vi "Read_Image(Batch).vi"(5 "mBatch":i32, 6 "PreProcessing_Options":T1={"DS_Name"="", "Input_Dims"={"C"=0, "H"=224, "W"=224}, "Center Crop Size"=-1, "Interpolation Type"=1, "Multi-Stage_DownSample?"=FALSE, "Dataset_Stats"={"means"={"R"=0.5385, "G"=0.5348, "B"=0.551}, "stds"={"R"=0.3673, "G"=0.3673, "B"=0.3505}}} {"Dataset_Stats"."stds"."R" format="%#_3g"; "Dataset_Stats"."stds"."G" format="%#_3g"; "Dataset_Stats"."stds"."B" format="%#_3g"; "Dataset_Stats"."means"."R" format="%#_3g"; "Dataset_Stats"."means"."G" format="%#_3g"; "Dataset_Stats"."means"."B" format="%#_3g"; "Interpolation Type" items=["Zero Order", "Bi-Linear", "Quadratic", "Cubic Spline"]}, 8 "error in":errorcluster, 9 "index":i32, 11 "Array":path[][](array[path])) -> (0 "error out":errorcluster, 2 "dT_Img_Read":dbl format="%0.2f", 3 "Image(Batch) Out":sgl[][][][](array[numeric]))   [LabVIEW 2020]
uses:
  <vilib>/Analysis/NI_AALBase.lvlib
  <vilib>/Analysis/baseanly.llb/Mean (DBL).vi
  <vilib>/Ngene/DeepLTK Anomaly Detection Addon/DeepLTK_Anomaly_Detection_Addon/API/Controls/NNPC_DS_Stats.ctl
  <vilib>/Ngene/DeepLTK Anomaly Detection Addon/DeepLTK_Anomaly_Detection_Addon/DeepLTK_Anomaly_Detection_Addon.lvlib
  <vilib>/Ngene/Deep Learning Toolkit/Toolkit/NN_Data/API/NN_Dims(C,H,W).ctl
  <vilib>/Ngene/Deep Learning Toolkit/Toolkit/Deep_Learning_Toolkit_by_Ngene.lvlib
  <vilib>/Ngene/DeepLTK Anomaly Detection Addon/DeepLTK_Anomaly_Detection_Addon/API/Controls/NNPC_PreProcessing_Options.ctl
  <vilib>/Ngene/DeepLTK Anomaly Detection Addon/DeepLTK_Anomaly_Detection_Addon/API/Controls/Image_Stats_RGB.ctl
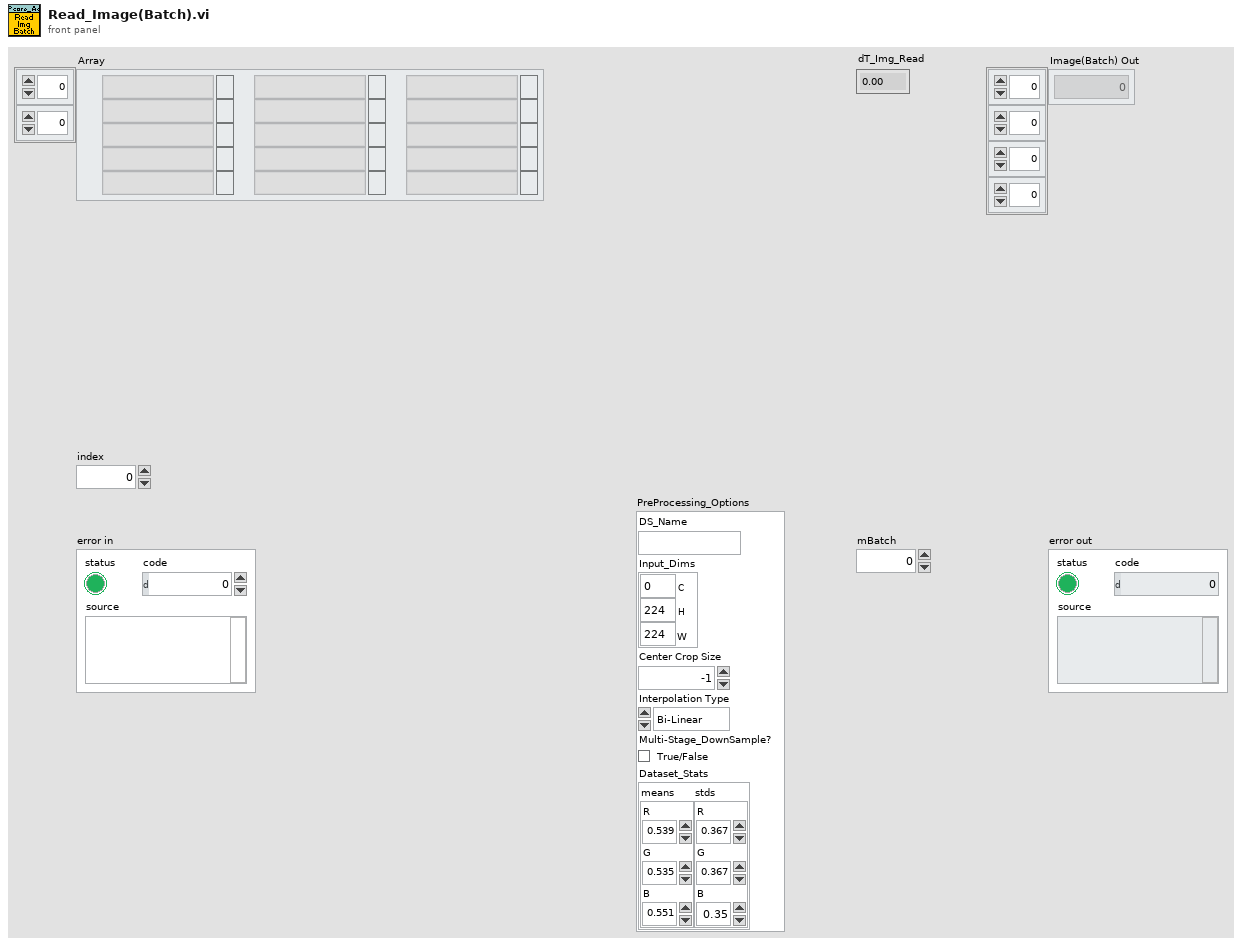
[diagram p1: front panel]
types:
  T1 = typedef "DeepLTK_Anomaly_Detection_Addon.lvlib/NNPC_PreProcessing_Options.ctl" = cluster{"DS_Name":string, "Input_Dims":T2, "Center Crop Size":i32, "Interpolation Type":u32, "Multi-Stage_DownSample?":bool, "Dataset_Stats":T3}
  T2 = typedef "Deep_Learning_Toolkit_by_Ngene.lvlib/NN_Dims(C,H,W).ctl" = cluster{"C":i32, "H":i32, "W":i32}
  T3 = typedef "DeepLTK_Anomaly_Detection_Addon.lvlib/NNPC_DS_Stats.ctl" = cluster{"means":T4, "stds":T4}
  T4 = typedef "DeepLTK_Anomaly_Detection_Addon.lvlib/Image_Stats_RGB.ctl" = cluster{"R":sgl, "G":sgl, "B":sgl}
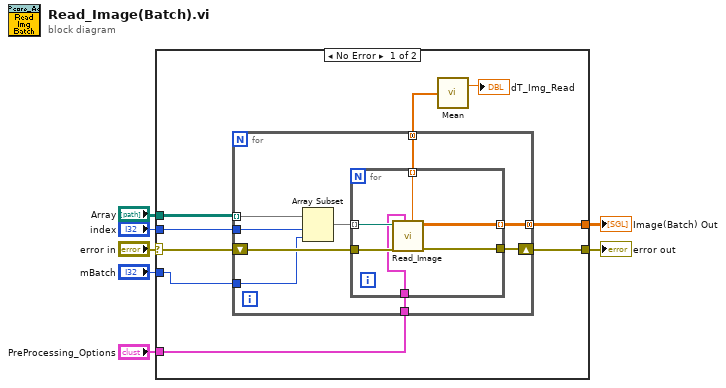
[diagram p0: block diagram]
diagram:
  n1 = case shown="No Error" "error in" {
    selector: "error in" -> [w9 w32]
    tunnel: [w16 _] -> w7
    tunnel: [w15 w32] -> w6
    tunnel: "Array" -> [w14 _]
    tunnel: "PreProcessing_Options" -> [w13 _]
    tunnel: "index" -> [w12 _]
    tunnel: "mBatch" -> [w8 _]
    frame No Error {
      n2 = for {
        tunnel: [w24] -> w11 mode=concatenating
        tunnel: w14 -> [w19] mode=indexing
        tunnel: [w23] -> w16 mode=concatenating
        tunnel: w13 -> [w21]
        shift-right: [w22] -> w15
        shift-left: w9 -> [w25]
        tunnel: w12 -> [w18]
        tunnel: w8 -> [w17]
        n3 = Array Subset(array=w19, index=w18, length=w17) -> (w20:path[])
        n4 = for {
          tunnel: w25 -> [w31]
          tunnel: [w30] -> w24 mode=indexing
          tunnel: w20 -> [w29] mode=indexing
          tunnel: [w28] -> w23 mode=indexing
          tunnel: [w27] -> w22
          tunnel: w21 -> [w26]
          n5 = call "Read_Image.vi"("PreProcessing_Options"=w26, "error in"=w31, "Img Path"=w29) -> ("error out"=w27:errorcluster, "Image Out"=w28:sgl[][][], "dT_Img_Read"=w30:dbl)  [unwired: 5 in, 1 out]
        }
      }
      n6 = call-poly <vilib>:"Mean.vi"("X"=w11) -> ("mean"=→"dT_Img_Read":dbl)  [unwired: 1 out]
    }
    frame Error {
    }
  }
  "Image(Batch) Out" <- w7
  "error out" <- w6
